vi "Mouse Up.vi"(8 "error in (no error)":errorcluster, 10 "Point":T1, 11 "Circle in":refnum<class "Circle.lvclass">) -> (0 "error out":errorcluster, 3 "Circle out":refnum<class "Circle.lvclass">)   [LabVIEW 2018, in "Circle.lvclass"]
doc: "A method for specifying how a circle reacts on a mouse up event"
uses:
  Circle.lvclass
  <vilib>/Utility/miscctls.llb/LVPoint32TypeDef.ctl
  Circle.lvclass/Circle.ctl
  Ellipse/Ellipse.lvclass
  Graphics Object/Graphics Object.lvclass
panel:
  # "expressionflow.com"
  # "Copyright (c) 2008 Tomi Maila. All rights reserved."
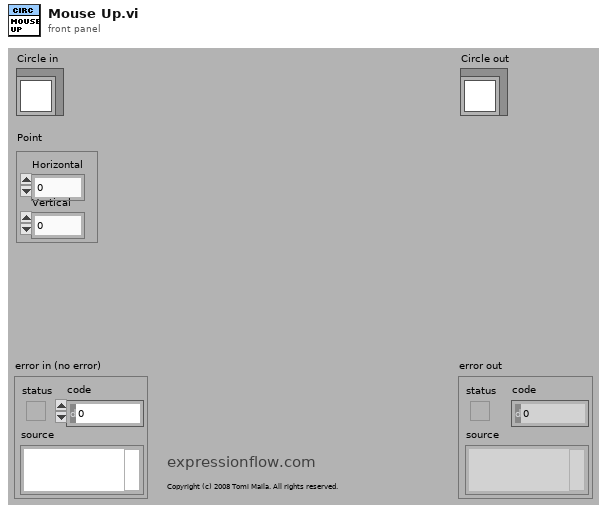
[diagram p1: front panel]
types:
  T1 = typedef "LVPoint32TypeDef.ctl" = cluster{"Horizontal":i32, "Vertical":i32}
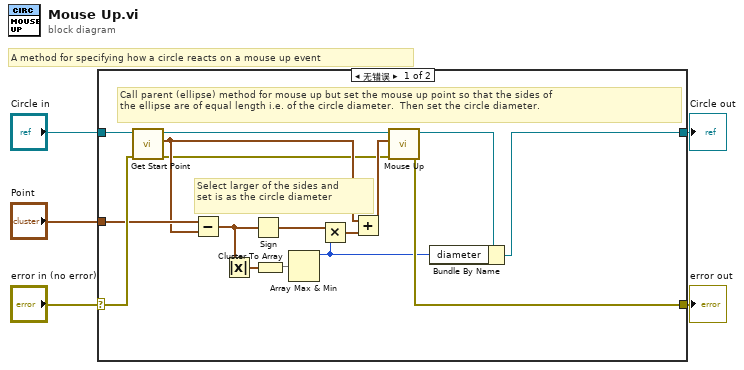
[diagram p0: block diagram]
diagram:
  # "A method for specifying how a circle reacts on a mouse up event"
  n1 = case shown="无错误" "error in (no error)" {
    selector: "error in (no error)" -> [w20 w22]
    tunnel: [w19 w22] -> w4
    tunnel: [w7 w23] -> w2
    tunnel: "Circle in" -> [w21 w23]
    tunnel: "Point" -> [w17 _]
    frame No Error {
      # "Select larger of the sides and \nset is as the circle diameter"
      # "Call parent (ellipse) method for mouse up but set the mouse up point so that the sides of \nthe ellipse are of equal length i.e. of the circle diameter.  Then set the circle diameter."
      n2 = call "Get Start Point.vi"("error in (no error)"=w20, "Graphics Object.lvclass in"=w21) -> ("error out"=w9:errorcluster, "start point"=w11:cluster{"x":i16, "y":i16}, "Graphics Object.lvclass out"=w18:refnum<class "Circle.lvclass">)  [unwired: 7 in]
      n3 = Subtract(x=w17, y=w11) -> (x-y=w14:T1)
      n4 = Absolute Value(x=w14) -> (abs(x)=w16:T1)
      n5 = Sign(1:w14) -> (0:w13:T1)
      n6 = Cluster To Array(cluster=w16) -> (array=w15:i32[])
      n7 = Array Max & Min(array=w15) -> (max value=w6:i32)  [unwired: 3 out]
      n8 = Multiply(x=w13, y=w6) -> (x*y=w12:T1)
      n9 = Add(x=w11, y=w12) -> (x+y=w10:T1)
      n10 = call-parent "Mouse Up.vi"("error in (no error)"=w9, "Point"=w10, "Ellipse in"=w18) -> ("error out"=w19:errorcluster, "Ellipse out"=w8:refnum<class "Circle.lvclass">)  [unwired: 7 in]
      n11 = Bundle By Name(cluster=w8, "diameter"=w6) -> (w7:refnum<class "Circle.lvclass">)
    }
    frame Error {
    }
  }
  "error out" <- w4
  "Circle out" <- w2
